vi "encodeUInt16.vi"(2 "Compress? (T)":bool=TRUE, 3 "UInt16":u16) -> (1 "MessagePack":u8[](array[numeric]) format="%.0x")   [LabVIEW 2015, in "MsgPack.lvlib"]
uses:
  MsgPack.lvlib
  SubVis/encodeFixedInt.vi
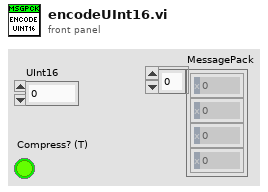
[diagram p1: front panel]
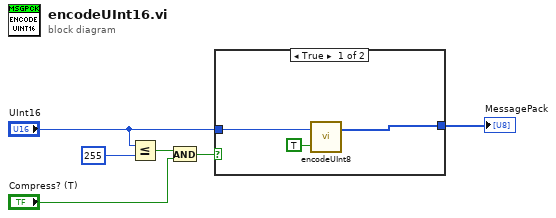
[diagram p0: block diagram]
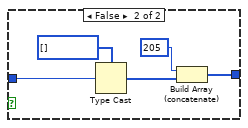
[diagram p2: hidden frame]
diagram:
  n1 = Less Or Equal?(x="UInt16", y=u16 255) -> (x <= y?=w4:bool)
  n2 = And(x=w4, y="Compress? (T)") -> (x .and. y?=w3:bool)
  n3 = case shown="True" w3 {
    tunnel: [w9 w14] -> w6
    tunnel: "UInt16" -> [w8 w10]
    frame True {
      n4 = call "encodeUInt8.vi"("Compress? (T)"=TRUE ("Compress"), "UInt8"=w8) -> ("MessagePack"=w9:u8[])  [unwired: 1 in]
    }
    frame False {
      n5 = Type Cast(type=u8[] [], x=w10) -> (*(type *) &x=w11:u8[])
      n6 = Build Array (concatenate)(u8 205, w11) -> (w14:u8[])
    }
  }
  "MessagePack" <- w6
